vi "Private Constants.vi"() -> ()   [LabVIEW 2016, in "AssertEngine.lvlib" / "AssertEngine.lvclass"]
uses:
  AssertEngine.lvclass
panel:
  in  "Tab Control":enum32{"Assert Attribute Identifiers", "Page 2"}(tab)
  in  "Build Timestamp":string="Timestamp"
  in  "Assert Name":string="Name"
  in  "Data Type":string="Data Type"
  in  "Assert VI UID":string="Assert VI UID"
  in  "Assert Builder":string="Assert Builder"
  in  "Assert VI Name":string="Assert VI"
  in  "Calling VI Name":string="Calling VI"
  in  "Failure Action":string="Failure Action"
  in  "Eval String":string="Eval String"
  in  "Comment":string="Comment"
  in  "Status":string="Status"
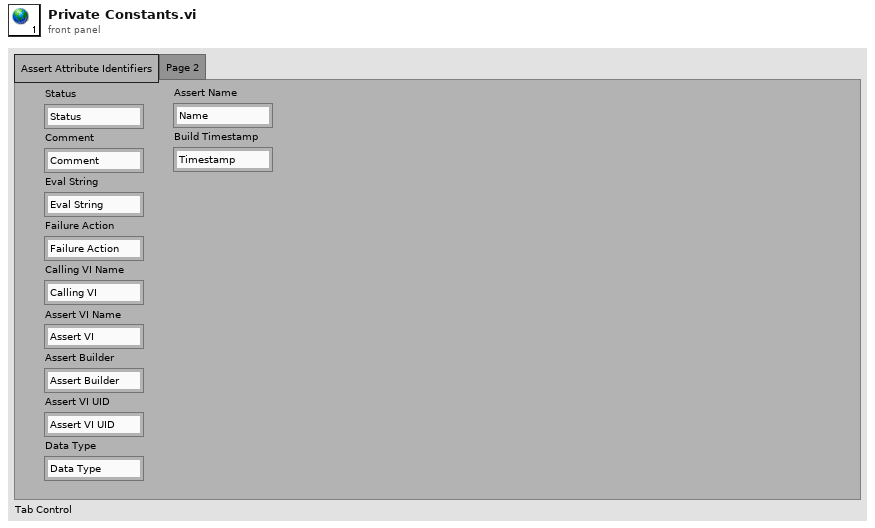
[diagram p1: front panel]
diagram:
